vi "Untitled 1.vi"() -> ()   [LabVIEW 2014]
panel:
  out "Numeric":dbl
  in  "stop":bool
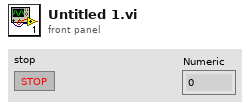
[diagram p1: front panel]
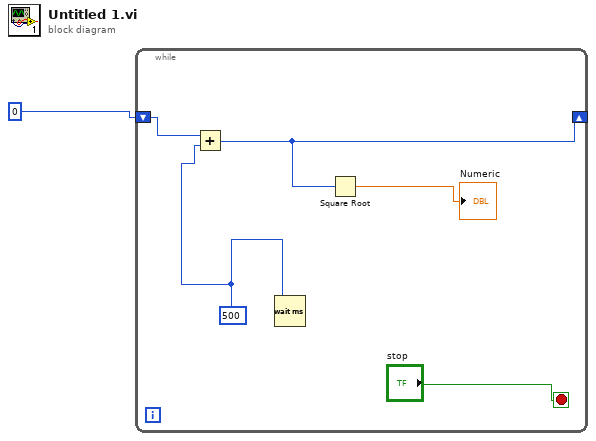
[diagram p0: block diagram]
diagram:
  n1 = while {
    shift-right: [w3] -> _
    shift-left: 0 -> [w4]
    stop <- "stop" stop-if-true
    w2 = 500
    n2 = Add(x=w4, y=w2) -> (x+y=w3:i32)
    n3 = Wait (ms)(milliseconds to wait=w2) -> ()  [unwired: 1 out]
    n4 = Square Root(x=w3) -> (sqrt(x)=→"Numeric":dbl)
  }
